vi "保存简单二进制文件.vi"() -> ()   [LabVIEW 2010]
panel:
  in  "文件（使用对话框）":path
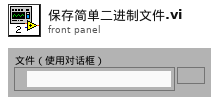
[diagram p1: front panel]
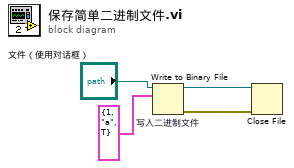
[diagram p0: block diagram]
diagram:
  n1 = Write to Binary File "写入二进制文件"(file (use dialog)="文件（使用对话框）", data=cluster{i32, string, bool} {1, "a", TRUE}) -> (refnum out=w4:refnum<file>, error out=w3:errorcluster)  [unwired: 4 in, 1 out]
  n2 = Close File(refnum=w4, error in=w3) -> ()  [unwired: 2 out]
